vi "sortGetConfig.vi"(11 "config data in":T1={"centerWavelength"=0.0, "chipHSpacing"=260.0, "chipHeight"=256.0, "chipName"="CCD30-11-1-275", "chipSerialNumber"="20091-22-21", "chipVSpacing"=260.0, "chipWidth"=1024.0, "deviceType"="HORIBA Scientific Syncerity", "fitParameters"=[0.0, 1.0, 0.0, 0.0, 0.0], "gains"=[{"info"="Best Dynamic Range", "token"=1}, {"info"="High Sensitivity", "token"=2}, {"info"="High Light", "token"=0}], "hardwareAvgAvailable"=FALSE, "lineScan"=FALSE, "productId"="13", "serialNumber"="Camera SN:  2244", "signals"=[{"events"=[{"name"="Ready For Trigger", "token"=1, "types"=[{"name"="TTL Active Low", "token"=1}, {"name"="TTL Active High", "token"=0}]}, {"name"="Shutter Open", "token"=3, "types"=[{"name"="TTL Active Low", "token"=1}, {"name"="TTL Active High", "token"=0}]}, {"name"="Reserved-DO NOT USE", "token"=2, "types"=[{"name"="TTL Active Low", "token"=1}, {"name"="TTL Active High", "token"=0}]}, {"name"="Start Experiment", "token"=0, "types"=[{"name"="TTL Active Low", "token"=1}, {"name"="TTL Active High", "token"=0}]}], "name"="Signal Output", "token"=0}], "speeds"=[{"info"=" 1 MHz       ", "token"=1}, {"info"="500 kHz Wrap", "token"=127}, {"info"=" 1 MHz Ultra ", "token"=2}, {"info"="45 kHz       ", "token"=0}], "supportedFeatures"={"cf_3PositionSlit"=FALSE, "cf_CMOSOffsetCorrection"=FALSE, "cf_Cleaning"=TRUE, "cf_DSP"=FALSE, "cf_DSPBin2X"=FALSE, "cf_DelayAfterTrigger"=FALSE, "cf_Delays"=FALSE, "cf_EMCCD"=FALSE, "cf_EShutter"=FALSE, "cf_HDR"=FALSE, "cf_Image"=TRUE, "cf_MemorySlots"=TRUE, "cf_Metadata"=FALSE, "cf_MultipleExposeTimes"=FALSE, "cf_MultipleSensors"=FALSE, "cf_PulseSummation"=FALSE, "cf_ROIs"=TRUE, "cf_Signals"=TRUE, "cf_Spectra"=TRUE, "cf_TriggerQualifier"=FALSE, "cf_Triggers"=TRUE}, "triggers"=[{"events"=[{"name"="Each - For Each Acq", "token"=1, "types"=[{"name"="TTL Rising  Edge", "token"=1}, {"name"="TTL Falling Edge", "token"=0}]}, {"name"="Once - Start All", "token"=0, "types"=[{"name"="TTL Rising  Edge", "token"=1}, {"name"="TTL Falling Edge", "token"=0}]}], "name"="Trigger Input", "token"=0}], "version"="Syncerity Ver 1.001.7.1"}) -> (3 "config data out":T1)   [LabVIEW 2023, in "CCD.lvclass"]
uses:
  CCD.lvclass
  GetConfig.ctl
  Gain.ctl
  Signal.ctl
  Event.ctl
  Type.ctl
  Speed.ctl
  SupportedFeatures.ctl
  Trigger.ctl
  CCD.lvclass/CCD.ctl
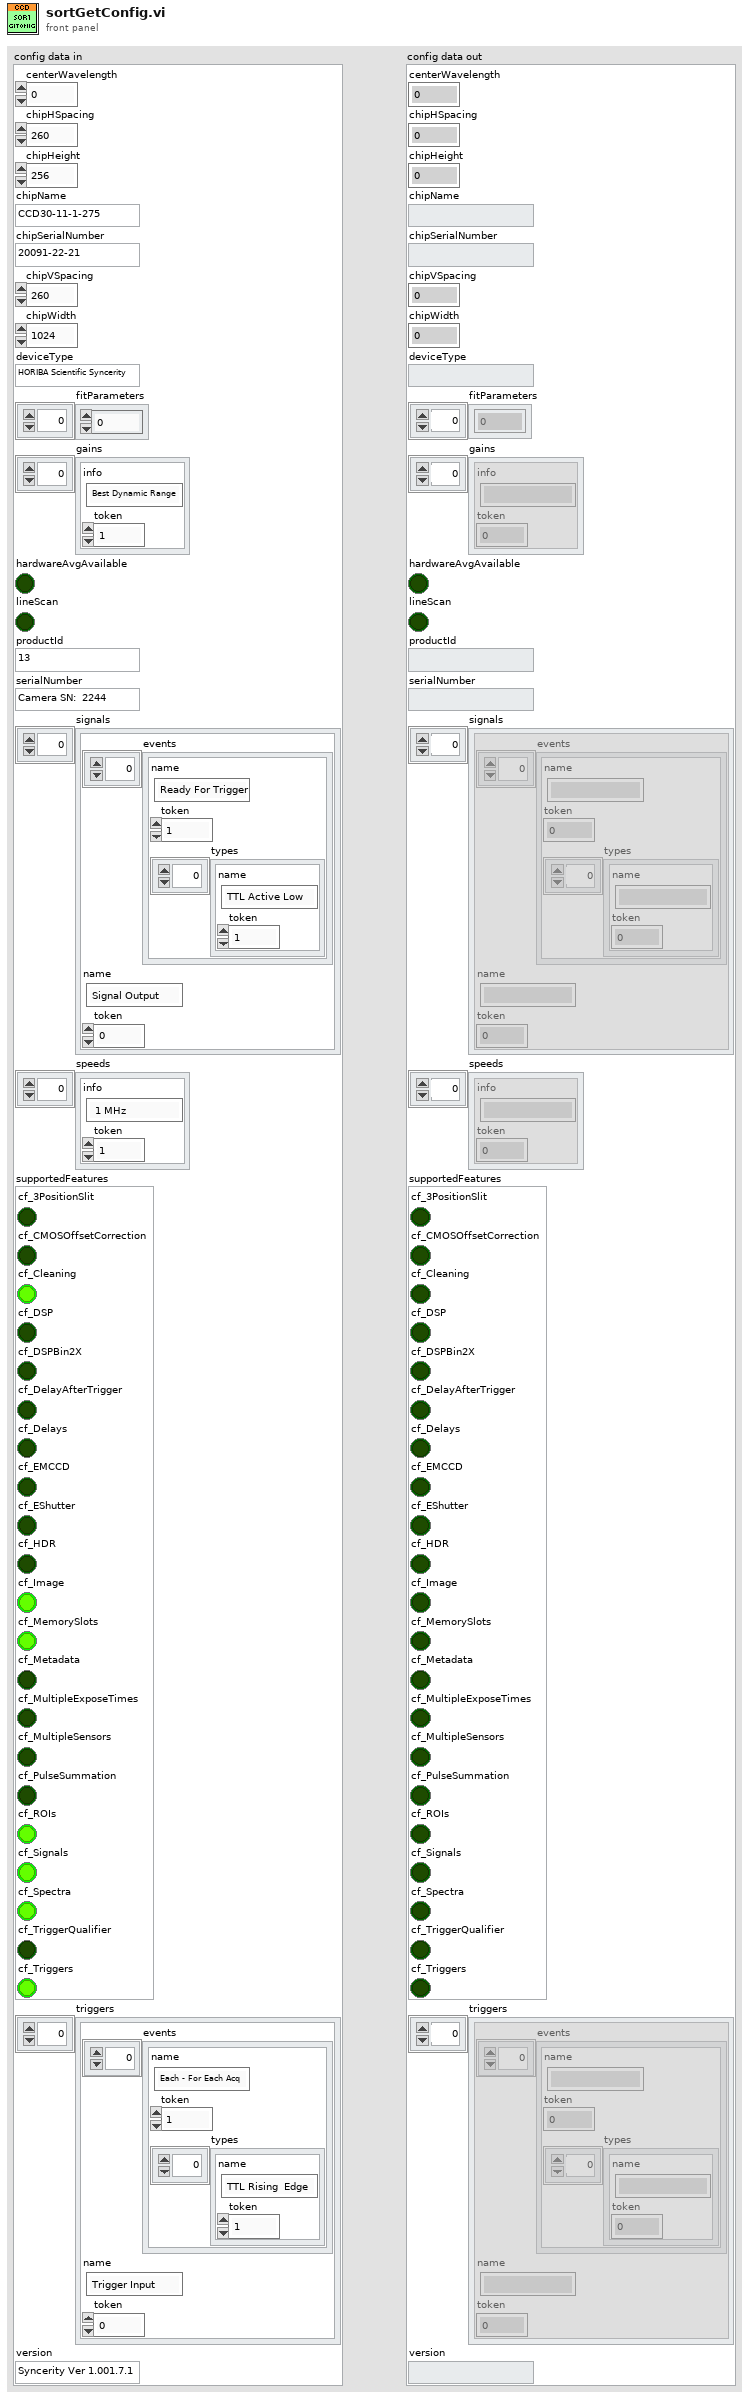
[diagram p1: front panel]
types:
  T1 = typedef "CCD.lvclass/GetConfig.ctl" = cluster{"centerWavelength":dbl, "chipHSpacing":dbl, "chipHeight":dbl, "chipName":string, "chipSerialNumber":string, "chipVSpacing":dbl, "chipWidth":dbl, "deviceType":string, "fitParameters":dbl[], "gains":T2[], "hardwareAvgAvailable":bool, "lineScan":bool, "productId":string, "serialNumber":string, "signals":T3[], "speeds":T6[], "supportedFeatures":T7, "triggers":T8[], "version":string}
  T2 = typedef "CCD.lvclass/Gain.ctl" = cluster{"info":string, "token":i32}
  T3 = typedef "CCD.lvclass/Signal.ctl" = cluster{"events":T4[], "name":string, "token":i32}
  T4 = typedef "CCD.lvclass/Event.ctl" = cluster{"name":string, "token":i32, "types":T5[]}
  T5 = typedef "CCD.lvclass/Type.ctl" = cluster{"name":string, "token":i32}
  T6 = typedef "CCD.lvclass/Speed.ctl" = cluster{"info":string, "token":i32}
  T7 = typedef "CCD.lvclass/SupportedFeatures.ctl" = cluster{"cf_3PositionSlit":bool, "cf_CMOSOffsetCorrection":bool, "cf_Cleaning":bool, "cf_DSP":bool, "cf_DSPBin2X":bool, "cf_DelayAfterTrigger":bool, "cf_Delays":bool, "cf_EMCCD":bool, "cf_EShutter":bool, "cf_HDR":bool, "cf_Image":bool, "cf_MemorySlots":bool, "cf_Metadata":bool, "cf_MultipleExposeTimes":bool, "cf_MultipleSensors":bool, "cf_PulseSummation":bool, "cf_ROIs":bool, "cf_Signals":bool, "cf_Spectra":bool, "cf_TriggerQualifier":bool, "cf_Triggers":bool}
  T8 = typedef "CCD.lvclass/Trigger.ctl" = cluster{"events":T4[], "name":string, "token":i32}
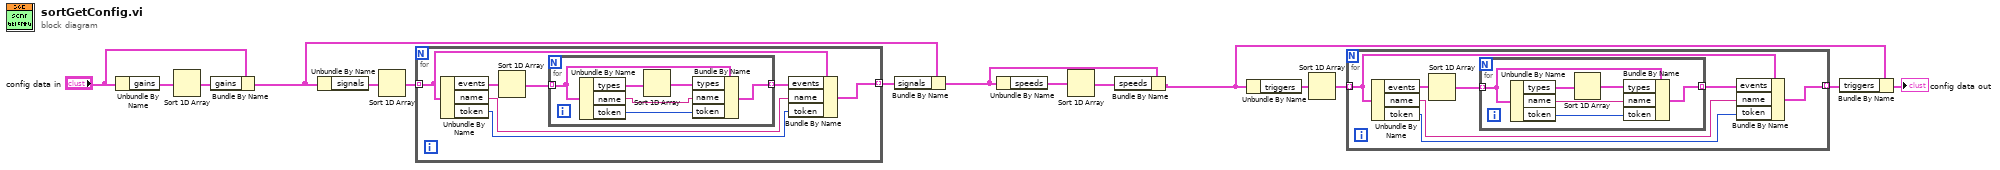
[diagram p0: block diagram]
diagram:
  n1 = Unbundle By Name("config data in") -> ("gains"=w14:T2[])
  n2 = Sort 1D Array(array=w14) -> (sorted array=w15:T2[])
  n3 = Bundle By Name(cluster="config data in", "gains"=w15) -> (w10:T1)
  n4 = Unbundle By Name(w10) -> ("signals"=w12:T3[])
  n5 = Sort 1D Array(array=w12) -> (sorted array=w11:T3[])
  n6 = for {
    tunnel: w11 -> [w20] mode=indexing
    tunnel: [w18] -> w9 mode=indexing
    n7 = Unbundle By Name(w20) -> ("events"=w22:T4[], "name"=w17:string, "token"=w16:i32)
    n8 = Sort 1D Array(array=w22) -> (sorted array=w21:T4[])
    n9 = for {
      tunnel: w21 -> [w26] mode=indexing
      tunnel: [w25] -> w19 mode=indexing
      n10 = Unbundle By Name(w26) -> ("types"=w28:T5[], "name"=w24:string, "token"=w23:i32)
      n11 = Sort 1D Array(array=w28) -> (sorted array=w27:T5[])
      n12 = Bundle By Name(cluster=w26, "types"=w27, "name"=w24, "token"=w23) -> (w25:T4)
    }
    n13 = Bundle By Name(cluster=w20, "events"=w19, "name"=w17, "token"=w16) -> (w18:T3)
  }
  n14 = Bundle By Name(cluster=w10, "signals"=w9) -> (w6:T1)
  n15 = Unbundle By Name(w6) -> ("speeds"=w7:T6[])
  n16 = Sort 1D Array(array=w7) -> (sorted array=w8:T6[])
  n17 = Bundle By Name(cluster=w6, "speeds"=w8) -> (w2:T1)
  n18 = Unbundle By Name(w2) -> ("triggers"=w5:T8[])
  n19 = Sort 1D Array(array=w5) -> (sorted array=w4:T8[])
  n20 = for {
    tunnel: w4 -> [w33] mode=indexing
    tunnel: [w31] -> w3 mode=indexing
    n21 = Unbundle By Name(w33) -> ("events"=w35:T4[], "name"=w30:string, "token"=w29:i32)
    n22 = Sort 1D Array(array=w35) -> (sorted array=w34:T4[])
    n23 = for {
      tunnel: w34 -> [w39] mode=indexing
      tunnel: [w38] -> w32 mode=indexing
      n24 = Unbundle By Name(w39) -> ("types"=w41:T5[], "name"=w37:string, "token"=w36:i32)
      n25 = Sort 1D Array(array=w41) -> (sorted array=w40:T5[])
      n26 = Bundle By Name(cluster=w39, "types"=w40, "name"=w37, "token"=w36) -> (w38:T4)
    }
    n27 = Bundle By Name(cluster=w33, "events"=w32, "name"=w30, "token"=w29) -> (w31:T8)
  }
  n28 = Bundle By Name(cluster=w2, "triggers"=w3) -> (→"config data out":T1)
